vi "Actor Core.vi"(8 "error in (no error)":errorcluster, 11 "Actor in":refnum<class "Actor1_GUI_G4_4.0.0.lvclass">) -> (0 "error out":errorcluster, 3 "Actor out":refnum<class "Actor.lvclass">)   [LabVIEW 2014, in "Actor1_GUI_G4_4.0.0.lvlib" / "Actor1_GUI_G4_4.0.0.lvclass"]
uses:
  <resource>/Framework/Providers/Open_GDS/ClassProviders/ActorFramework/4.0.0/Actor1_GUI_G4_4.0.0/Actor1_GUI_G4_4.0.0_Actor/Actor1_GUI_G4_4.0.0.lvclass
  <vilib>/ActorFramework/Actor/Actor.lvclass
panel:
  out "Waveform Graph":dynamicdata(graph)
  in  "Freq":dbl(slide)=10.1 scale=0.0..20.0
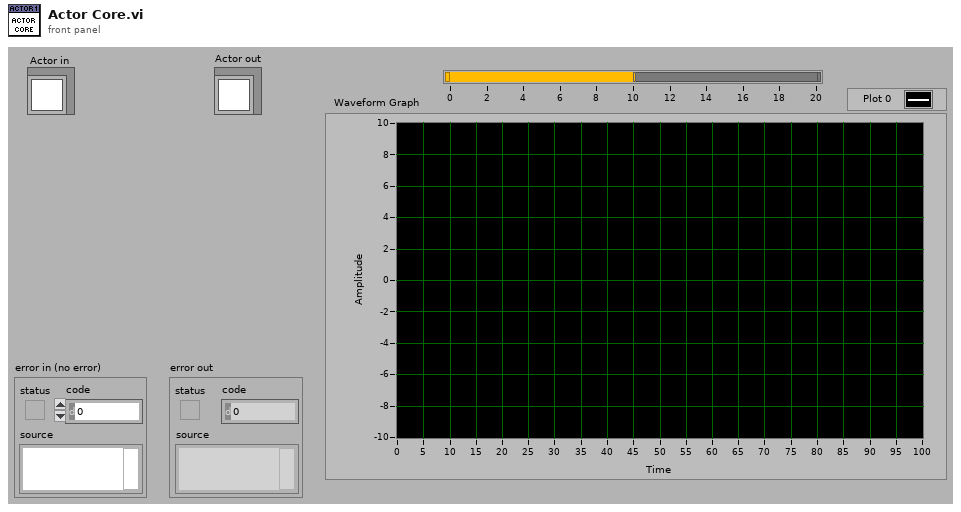
[diagram p1: front panel]
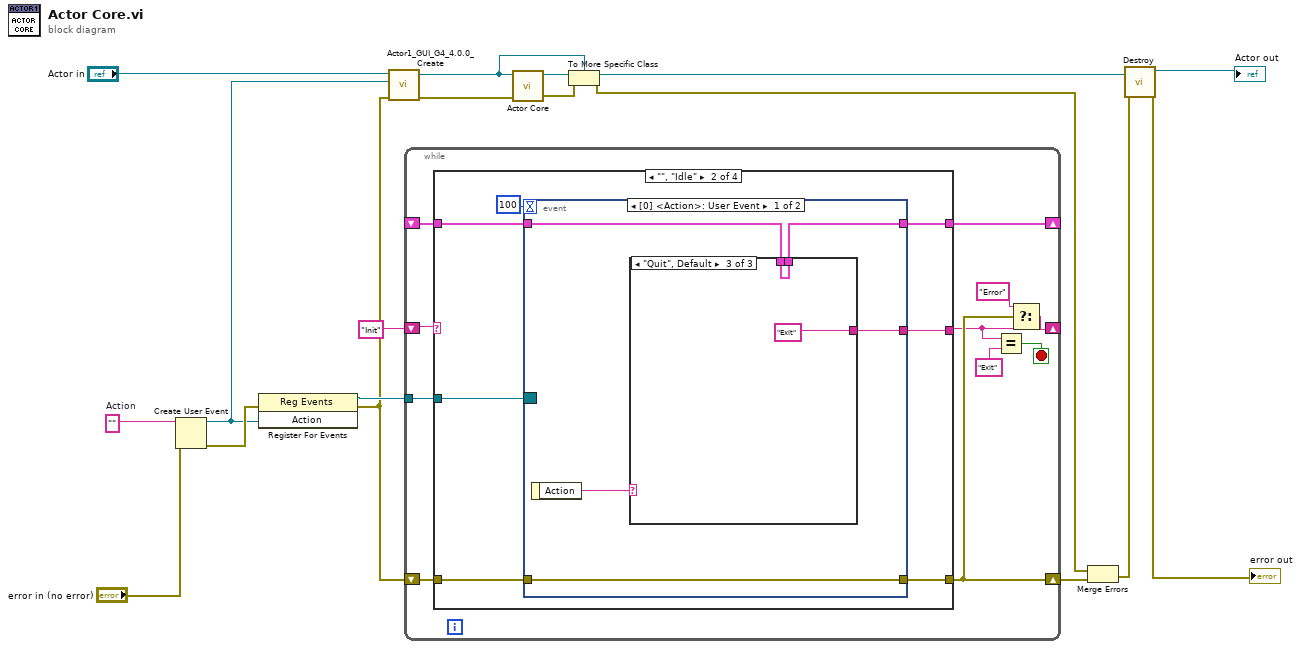
[diagram p0: block diagram]
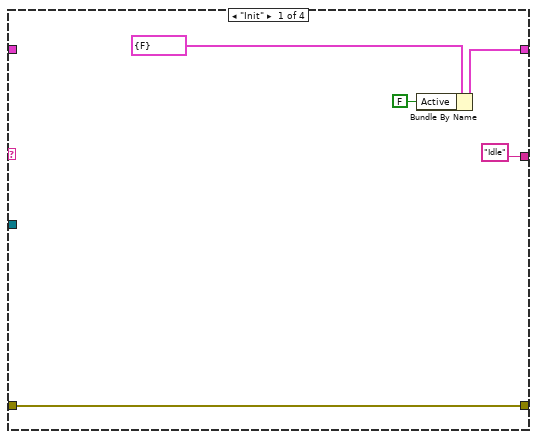
[diagram p2: hidden frame]
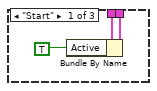
[diagram p3: hidden frame]
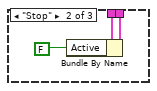
[diagram p4: hidden frame]
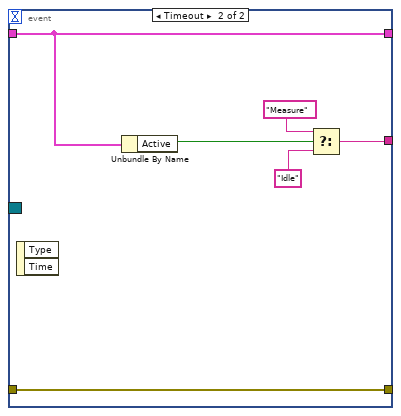
[diagram p5: hidden frame]
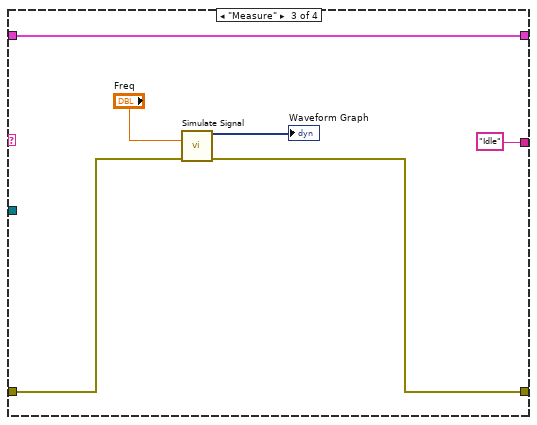
[diagram p6: hidden frame]
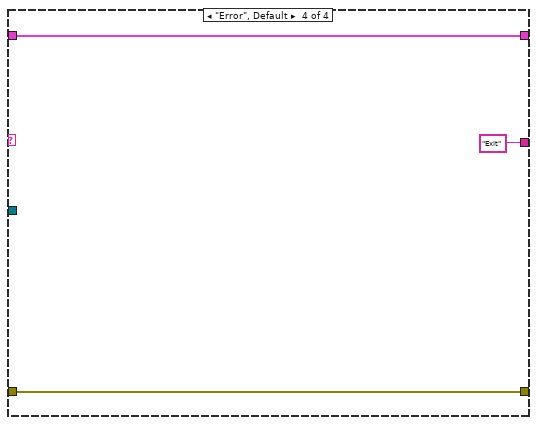
[diagram p7: hidden frame]
diagram:
  w1 = ""  # Action
  n1 = Create User Event(user event datatype=w1, error in="error in (no error)") -> (user event=w10:refnum<user-event>, error out=w15:errorcluster)
  n2 = register-events(error in=w15, w10) -> (reference out=w16:refnum<event-registration>, error out=w12:errorcluster)  [unwired: 1 in]
  n3 = call <resource>:"Actor1_GUI_G4_4.0.0_Create.vi"("error in (no error)"=w12, "LoopEvent"=w10, "reference in"="Actor in") -> ("error out"=w11:errorcluster, "reference out"=w8:refnum<class "Actor1_GUI_G4_4.0.0.lvclass">)  [unwired: 7 in]
  n4 = while {
    tunnel: w16 -> [w29]
    shift-right: [w24] -> _
    shift-left: "Init" -> [w28]
    shift-right: [w25] -> w14
    shift-left: w12 -> [w27]
    shift-right: [w21] -> _
    shift-left: _ -> [w20]
    stop <- w26 stop-if-true
    n5 = case shown="\"\", \"Idle\"" w28 {
      tunnel: w29 -> [_ w41 _ _]
      tunnel: ["Idle" w40 "Idle" "Exit" ("y")] -> w22
      tunnel: w27 -> [w33 w37 w61 w68]
      tunnel: [w33 w36 w62 w68] -> w25
      tunnel: [w30 w38 w64 w67] -> w21
      tunnel: w20 -> [_ w35 w64 w67]
      frame "Init" {
        n6 = Bundle By Name(cluster=cluster{"Active":bool} {"Active"=FALSE}, "Active"=FALSE) -> (w30:cluster{"Active":bool})
      }
      frame "", "Idle" {
        n7 = event shown="[0] <Action>: User Event" {
          selector: w41 -> [_ _]
          dyn-events: _ -> [_ _]
          timeout: 100 -> [_ _]
          tunnel: [w45 w55] -> w40
          tunnel: w35 -> [w44 w59]
          tunnel: [w43 w59] -> w38
          tunnel: w37 -> [w42 w60]
          tunnel: [w42 w60] -> w36
          event User Event {
            n8 = event-data() -> ("Action"=w46:string)  [unwired: 1 in]
            n9 = case shown="\"Quit\", Default" w46 {
              tunnel: [_ _ "Exit" ("y")] -> w45
              tunnel: w44 -> [w49 w52 w53]
              tunnel: [w48 w51 w53] -> w43
              frame "Start" {
                n10 = Bundle By Name(cluster=w49, "Active"=TRUE) -> (w48:cluster{"Active":bool})
              }
              frame "Stop" {
                n11 = Bundle By Name(cluster=w52, "Active"=FALSE) -> (w51:cluster{"Active":bool})
              }
              frame "Quit", Default {
              }
            }
          }
          event Timeout {
            n12 = event-data() -> ()  [unwired: 1 in, 2 out]
            n13 = Unbundle By Name(w59) -> ("Active"=w58:bool)
            n14 = Select(t="Measure", s=w58, f="Idle") -> (s? t:f=w55:string)
          }
        }
      }
      frame "Measure" {
        n15 = call "Simulate Signal"("Frequency"="Freq", "error in (no error)"=w61) -> ("Sine with Uniform Noise"=→"Waveform Graph":dynamicdata, "error out"=w62:errorcluster)  [unwired: 12 in]
      }
      frame "Error", Default {
      }
    }
    n16 = Equal?(x=w22, y="Exit") -> (x = y?=w26:bool)
    n17 = Select(t="Error", s=w25, f=w22) -> (s? t:f=w24:string)
  }
  n18 = call-parent "Actor Core.vi"("error in"=w11, "Actor in"=w8) -> ("error out"=w7:errorcluster, "Actor out"=w9:refnum<class "Actor.lvclass">)  [unwired: 8 in]
  n19 = To More Specific Class(target class=w8, reference=w9, error in=w7) -> (specific class reference=w5:refnum<class "Actor1_GUI_G4_4.0.0.lvclass">, error out=w6:errorcluster)
  n20 = Merge Errors(w6, w14) -> (w4:errorcluster)
  n21 = call-dynamic "Destroy.vi"("error in (no error)"=w4, "reference in"=w5) -> ("error out"=→"error out":errorcluster, "reference out"=→"Actor out":refnum<class "Actor1_GUI_G4_4.0.0.lvclass">)  [unwired: 8 in]
